vi "Register Seq File Callback Refs.vi"(8 "error in (no error)":errorcluster, 11 "teststand-api in":refnum<class "teststand-api.lvclass">) -> (0 "error out":errorcluster, 3 "teststand-api out":refnum<class "teststand-api.lvclass">)   [LabVIEW 2014, in "teststand-api.lvlib" / "teststand-api.lvclass"]
uses:
  teststand-api.lvclass
  Callback References Argument--cluster.ctl
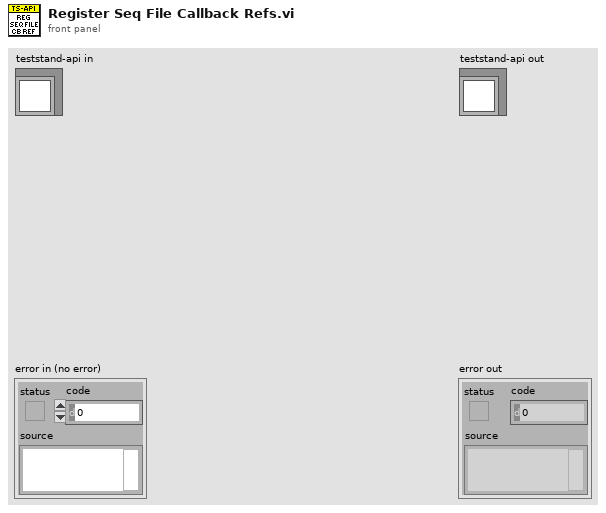
[diagram p1: front panel]
types:
  T1 = typedef "teststand-api.lvlib/teststand-api.lvclass/Callback References Argument--cluster.ctl" = cluster{"Sequence File Callback Ref":refnum<k27>}
  T2 = typedef "teststand-api.lvlib/teststand-api.lvclass/TS Controls Argument--cluster.ctl" = cluster{"Execution View":refnum<k7>, "Sequence View":refnum<k7>, "Report View":refnum<k7>}
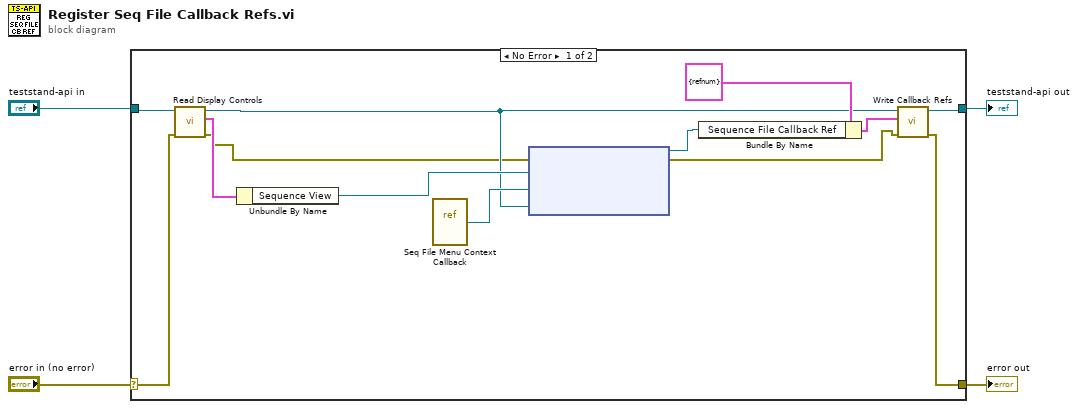
[diagram p0: block diagram]
diagram:
  n1 = case shown="No Error" "error in (no error)" {
    selector: "error in (no error)" -> [w9 w19]
    tunnel: [w10 w19] -> w3
    tunnel: [w14 w18] -> w1
    tunnel: "teststand-api in" -> [w17 w18]
    frame No Error {
      n2 = call-dynamic "Read Display Controls.vi"("error in (no error)"=w9, "teststand-api in"=w17) -> ("error out"=w6:errorcluster, "Visible Controls"=w16:T2, "teststand-api out"=w7:refnum<class "teststand-api.lvclass">)  [unwired: 7 in]
      n3 = Unbundle By Name(w16) -> ("Sequence View"=w15:refnum<k7>)
      n4 = vi-ref "Seq File Menu Context Callback.vi"() -> ("vi reference"=w8:refnum<vi>)
      n5 = node(w6, w15, w8, w7) -> (w11:refnum<k27>, w5:errorcluster)  [unwired: 1 in]
      n6 = Bundle By Name(cluster=T1 {"Sequence File Callback Ref"=refnum} ("Callback Refs"), "Sequence File Callback Ref"=w11) -> (w12:T1)
      n7 = call-dynamic "Write Callback Refs.vi"("error in (no error)"=w5, "Callback Refs"=w12, "teststand-api in"=w7) -> ("error out"=w10:errorcluster, "teststand-api out"=w14:refnum<class "teststand-api.lvclass">)  [unwired: 7 in]
    }
    frame Error {
    }
  }
  "error out" <- w3
  "teststand-api out" <- w1
